vi "Execute Clean Up Button.vi"(6 "Mouse Position":T1, 8 "User VI Ref":refnum<vi>, 9 "Menu Item Tag Suffix":string, 10 "Remaining Items":refnum<vi>[](array[refnum]), 11 "Affected Items":T2) -> (0 "Fail transaction?":bool)   [LabVIEW 2025]
doc: "This VI is part of a plug-in for modifying the LabVIEW shortcut menus. This is the execute VI which is called when the shortcut menu is chosen by the user. It performs the action of the selected menu item."
uses:
  Clean Up Button.ctl
  <vilib>/Utility/miscctls.llb/LVPositionTypeDef.ctl
panel:
  out "error out":errorcluster
  # "All controls on this panel except \"Affected Items\" have been locked to prevent accidental edits. Changing the control names or types, other than the elements of the \"Affected Items\" cluster will make the VI unusable as a menu plugin.\n\nSee Context Help for each control for details about its use."
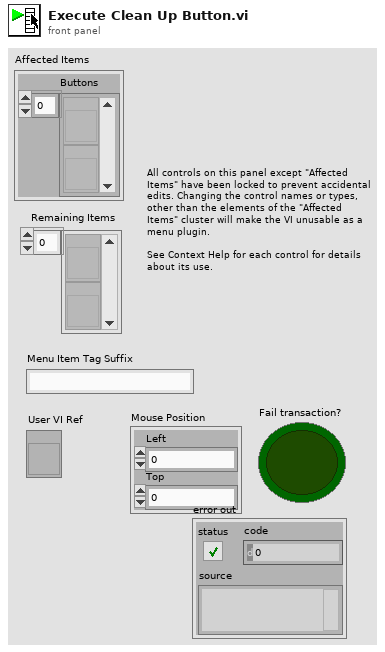
[diagram p1: front panel]
types:
  T1 = typedef "LVPositionTypeDef.ctl" = cluster{"Left":i32, "Top":i32}
  T2 = typedef "Clean Up Button.ctl" = cluster{"Buttons":refnum<vi>[]}
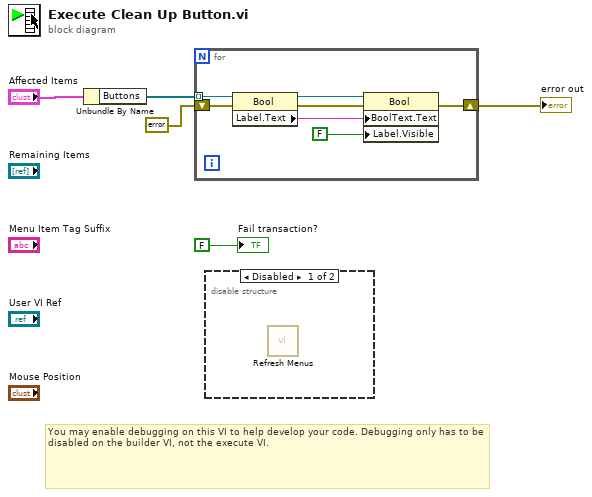
[diagram p0: block diagram]
diagram:
  # "You may enable debugging on this VI to help develop your code. Debugging only has to be disabled on the builder VI, not the execute VI."
  n1 = Unbundle By Name("Affected Items") -> ("Buttons"=w3:refnum<vi>[])
  n2 = for {
    tunnel: w3 -> [w12] mode=indexing
    shift-right: [w7] -> w1
    shift-left: errorcluster {"status"=FALSE, "code"=0, "source"=""} ("error out") -> [w6]
    n3 = property class="Bool"(reference=w12, error in=w6) -> (reference out=w10:refnum<vi>, error out=w9:errorcluster, "Label.Text"=w11:string)
    n4 = property class="Bool"(reference=w10, error in=w9, "BoolText.Text"=w11, "Label.Visible"=FALSE) -> (error out=w7:errorcluster)  [unwired: 1 out]
  }
  "error out" <- w1
  n5 = disable-structure shown="Disabled" {
    frame Disabled {
      n6 = call <resource>:"Refresh Menus.vi"() -> ()  [unwired: 12 in]
    }
    frame Enabled {
    }
  }
  "Fail transaction?" <- FALSE ("Fail transaction?")
